vi "NF90 run delay.vi"(4 "i":i32, 6 "axis":T1, 8 "Error In":errorcluster, 9 "delay (ms)":u32, 10 "port number":refnum<visa-resource-name>, 11 "Connection ID":refnum<k5>) -> (0 "Error Out":errorcluster, 1 "Position":sgl format="%.2f", 2 "killed":bool, 3 "Connection ID out":refnum<k5>)   [LabVIEW 2015]
uses:
  Axis.ctl
  NF90 commands.ctl
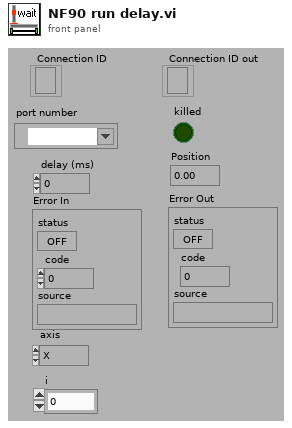
[diagram p1: front panel]
types:
  T1 = typedef "Axis.ctl" = enum16{"X", "Y", "Z"}
  T2 = typedef "NF90 commands.ctl" = enum16{"Index", "Speed", "Acceleration", "Backlash", "Quit", "Run", "Null indexes", "Verify status", "Clear program", "Computer Control", "Go", "Put Controller on Hold", "Position"}
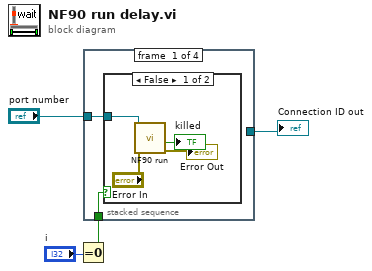
[diagram p0: block diagram]
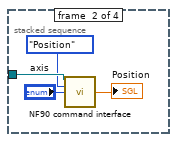
[diagram p3: hidden frame]
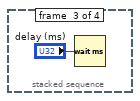
[diagram p4: hidden frame]
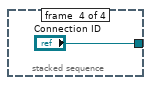
[diagram p5: hidden frame]
diagram:
  n1 = Equal To 0?(x="i") -> (x = 0?=w1:bool)
  n2 = stacked-sequence {
    tunnel: [_ _ _ "Connection ID"] -> w4
    tunnel: "port number" -> [w6 w14 _ _]
    tunnel: w1 -> [w5 _ _ _]
    frame #0 {
      n3 = case shown="False" w5 {
        tunnel: w6 -> [w10 _]
        frame False {
          n4 = call "NF90 run.vi"("Error In"="Error In", "port number in"=w10) -> ("Error Out"=→"Error Out":errorcluster, "killed"=→"killed":bool)  [unwired: 7 in, 1 out]
        }
        frame True {
        }
      }
    }
    frame #1 {
      n5 = call "NF90 command interface.vi"("port number in"=w14, "commands"=NF90_commands."Position", "axis"="axis") -> ("Position"=→"Position":sgl)  [unwired: 8 in, 4 out]
    }
    frame #2 {
      n6 = Wait (ms)(milliseconds to wait="delay (ms)") -> ()  [unwired: 1 out]
    }
    frame #3 {
    }
  }
  "Connection ID out" <- w4
